vi "LED Metronome.vi"() -> ()   [LabVIEW 2014]
panel:
  in  "stop":bool
  out "LED":bool
  in  "Blinks Per Minute":i32
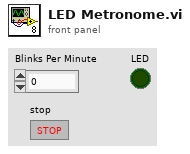
[diagram p1: front panel]
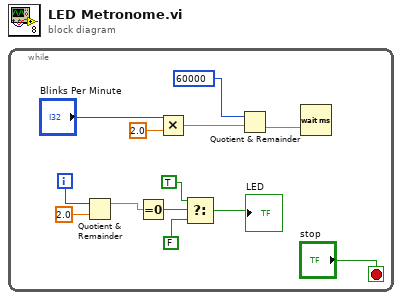
[diagram p0: block diagram]
diagram:
  n1 = while {
    i -> [w9]
    stop <- "stop" stop-if-true
    n2 = Quotient & Remainder(x=w9, y=2.0) -> (x-y*floor(x/y)=w7:dbl)  [unwired: 1 out]
    n3 = Equal To 0?(x=w7) -> (x = 0?=w8:bool)
    n4 = Multiply(x="Blinks Per Minute", y=2.0) -> (x*y=w1:dbl)
    n5 = Select(t=TRUE, s=w8, f=FALSE) -> (s? t:f=→"LED":bool)
    n6 = Quotient & Remainder(x=60000, y=w1) -> (floor(x/y)=w11:dbl)  [unwired: 1 out]
    n7 = Wait (ms)(milliseconds to wait=w11) -> ()  [unwired: 1 out]
  }
